vi "DAQmx(AI).TestLauncher.vi"() -> ()   [LabVIEW 2019, in "DAQmx(AI).lvclass"]
doc: "JKI State Machine Objects (SMO) 1.0.0.5\nJKI - JKI\nCopyright (c) 2016, JKI"
uses:
  DAQmx(AI).lvclass
  Typedefs/Scaling(MapRange)--Cluster.ctl
  Typedefs/InputConfiguration--Cluster.ctl
  Typedefs/Units -- Enum.ctl
  vi.lib/JKI/JKI SMO/SMO/Typedefs/SMOState --Enum.ctl
  C:/Users/Patrick/Documents/GitHub/Test (LV2019)/lv-venv/lv.lib/vi.lib/JKI/JKI SMO/SMO/SMO.lvclass
  Set Scaling (MapRange).vi
  vi.lib/JKI/JKI SMO/SMO/SMO.lvclass
panel:
  in  "TDMS File Path":path
  out "Waveform Chart":dbl(graph) caption="Waveform Graph"
  in  "Physical Channel":tag="SMO-Sim/ai0"
  out "Device Name":tag="SMO-Sim"
  out "Simulated":bool
  out "Device found":bool
  out "error out":errorcluster
  in  "Stop":bool
  # "Analog Input DAQmx Test Launcher"
  # "For instructions on how to use the JKI State Machine Objects, examples and video tutorials, visit:\nhttp://jki.net/state-machine-objects/\n\nJKI State Machine Objects™\nhttp://jki.net/state-machine-objects/\nCopyright (C) 2005-2016, JKI <info@jki.net>\nALL RIGHTS RESERVED"
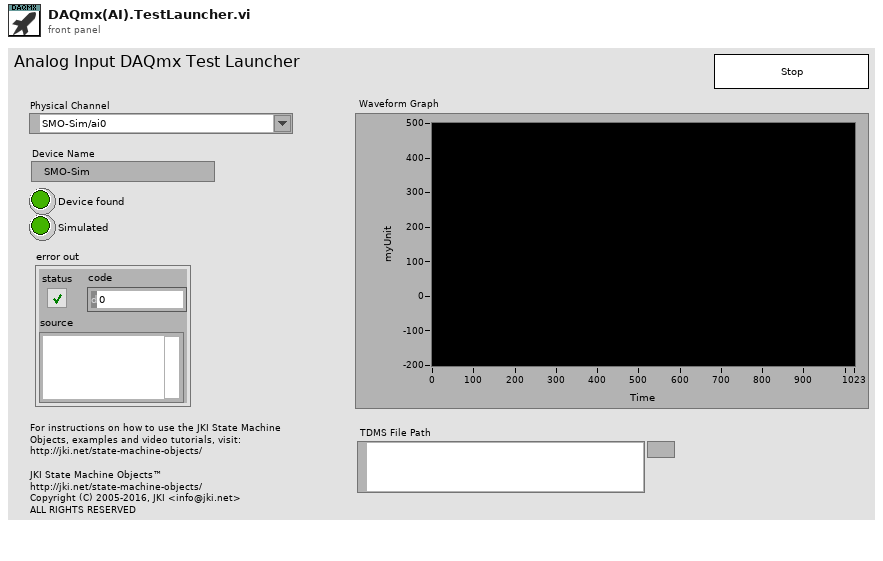
[diagram p1: front panel]
types:
  T1 = typedef "DAQmx(AI).lvclass/InputConfiguration--Cluster.ctl" = cluster{"input terminal":i32, "minimum value":dbl, "maximum value":dbl, "units":T2}
  T2 = typedef "DAQmx(AI).lvclass/Units -- Enum.ctl" = enum16{"Volts", "Amps", "Deg F", "Deg C", "Deg R", "Kelvins", "Strain", "Ohms", "Hz", "Seconds", "Meters", "Inches", "Degrees", "Radians", "Ticks", "g", "m/s^2", "m/s", "in/s", "Pascals", "Newtons", "Pounds", "kgf", "psi", "bar", "Nm", "oz-in", "lb-in", "lb-ft", "Volts/Volt", "mVolts/Volt", "From TEDS"}
  T3 = typedef "DAQmx(AI).lvclass/Scaling(MapRange)--Cluster.ctl" = cluster{"Minimum":dbl, "Maximum":dbl}
  T4 = typedef "DAQmx(AI).lvclass/PublicEvents--Cluster.ctl" = cluster{"Value Changed":refnum<user-event>, "Task Configuration":refnum<user-event>, "Scaling":refnum<user-event>}
  T5 = typedef "SMO.lvclass/Public Events.ctl" = cluster{"Error":refnum<user-event>, "State":refnum<user-event>, "Reserve State":refnum<user-event>}
  T6 = typedef "SMO.lvclass/SMOState --Enum.ctl" = enum16{"unknown", "Created", "Started", "Stopped"}
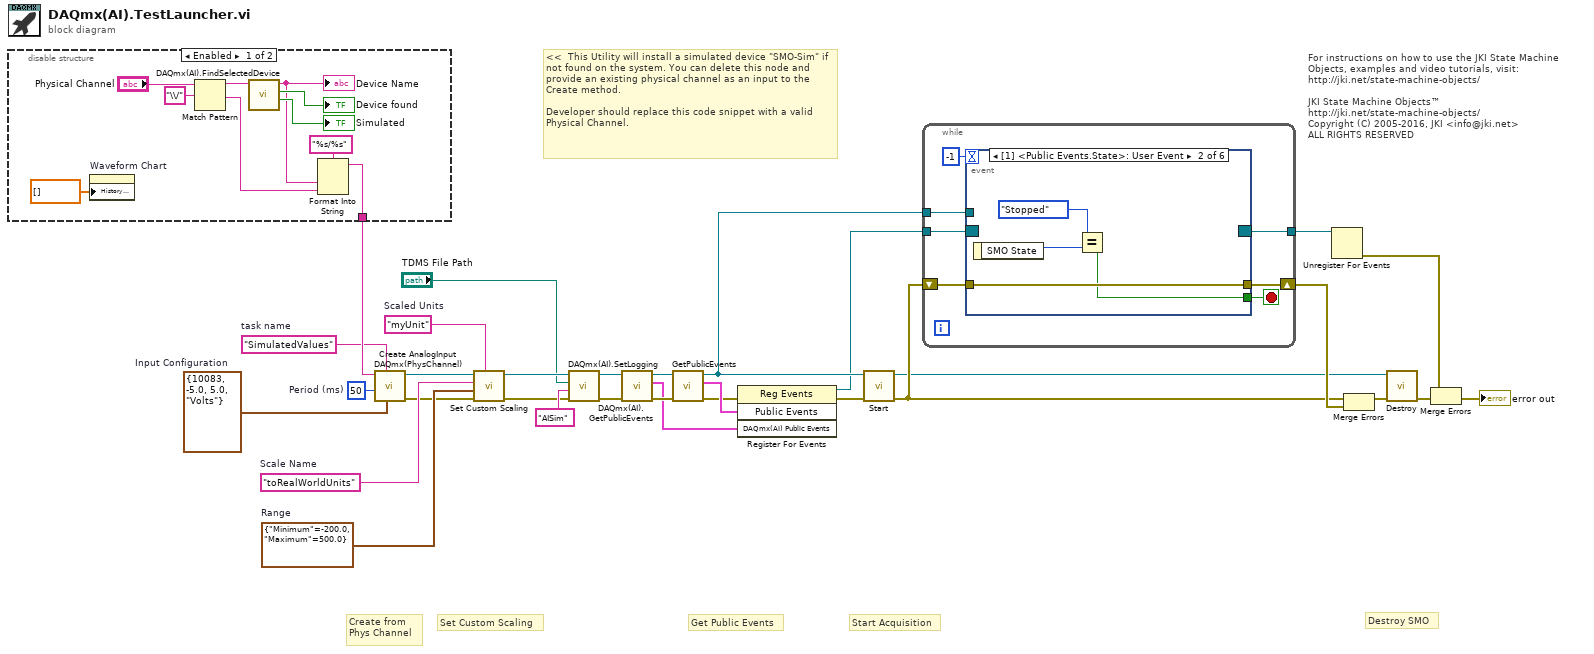
[diagram p0: block diagram]
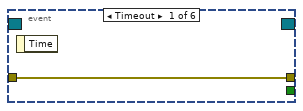
[diagram p3: hidden frame]
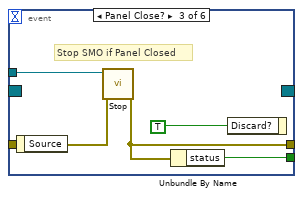
[diagram p4: hidden frame]
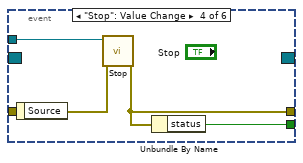
[diagram p5: hidden frame]
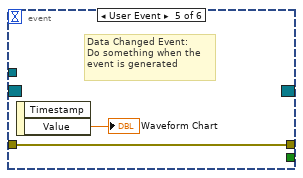
[diagram p6: hidden frame]
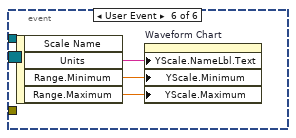
[diagram p7: hidden frame]
diagram:
  w1 = "SimulatedValues"  # task name
  w8 = T1 {"input terminal"=10083, "minimum value"=-5.0, "maximum value"=5.0, "units"=enum."Volts"}  # Input Configuration
  w9 = "myUnit"  # Scaled Units
  w11 = T3 {"Minimum"=-200.0, "Maximum"=500.0}  # Range
  w12 = "toRealWorldUnits"  # Scale Name
  w15 = i64 50  # Period (ms)
  # "Create from\nPhys Channel"
  # "Set Custom Scaling"
  # "<<  This Utility will install a simulated device \"SMO-Sim\" if not found on the system. You can delete this node and provide an existing physical channel as an input to the Create method.\n\nDeveloper should replace this code snippet with a valid Physical Channel."
  # "For instructions on how to use the JKI State Machine Objects, examples and video tutorials, visit:\nhttp://jki.net/state-machine-objects/\n\nJKI State Machine Objects™\nhttp://jki.net/state-machine-objects/\nCopyright (C) 2005-2016, JKI <info@jki.net>\nALL RIGHTS RESERVED"
  # "Get Public Events"
  # "Start Acquisition"
  # "Destroy SMO"
  n1 = disable-structure shown="Enabled" {
    disable-tunnel: [w33 _] -> w14
    frame Enabled {
      n2 = property on="Waveform Chart" class="WFChart (strict)"("History Data"=dbl[] []) -> ()  [unwired: 2 in, 2 out]
      n3 = Match Pattern(string="Physical Channel", regular expression="\\/") -> (before substring=w37:string, after substring=w35:string)  [unwired: 1 in, 2 out]
      n4 = call "DAQmx(AI).FindSelectedDevice.vi"("Device Name"=w37) -> ("Simulated"=→"Simulated":bool, "Device found"=→"Device found":bool, "ActiveDev"=w36:tag)  [unwired: 7 in, 1 out]
      "Device Name" <- w36
      n5 = Format Into String(format string="%s/%s", w36, w35) -> (resulting string=w33:string)  [unwired: 2 in, 1 out]
    }
    frame Disabled {
    }
  }
  n6 = call "Create AnalogInput DAQmx(PhysChannel).vi"("Input Configuration"=w8, "task name"=w1, "Period (ms)"=w15, "DAQmx Physical Channel"=w14) -> ("error out"=w10:errorcluster, "Subsystem out"=w13:refnum<class "DAQmx(AI).lvclass">)  [unwired: 5 in, 1 out]
  n7 = call-poly "Set Custom Scaling.vi"("Scaled Units"=w9, "error in (no error)"=w10, "Map Range"=w11, "Scale Name"=w12, "DAQmx(AI) in"=w13) -> ("error out"=w4:errorcluster, "DAQmx(AI) out"=w6:refnum<class "DAQmx(AI).lvclass">)  [unwired: 5 in]
  n8 = call "DAQmx(AI).SetLogging.vi"("error in (no error)"=w4, "Group Name"="AISim", "TDMS File Path"="TDMS File Path", "DAQmx(AI) in"=w6) -> ("error out"=w3:errorcluster, "DAQmx(AI) out"=w5:refnum<class "DAQmx(AI).lvclass">)  [unwired: 6 in]
  n9 = call "DAQmx(AI).GetPublicEvents.vi"("error in (no error)"=w3, "Subsystem"=w5) -> ("error out"=w18:errorcluster, "DAQmx(AI) Public Events"=w16:T4, "Subsystem out"=w17:refnum<class "DAQmx(AI).lvclass">)  [unwired: 7 in]
  n10 = call "GetPublicEvents.vi"("error in (no error)"=w18, "SMO"=w17) -> ("error out"=w20:errorcluster, "Public Events"=w21:T5, "SMO out"=w23:refnum<class "DAQmx(AI).lvclass">)  [unwired: 7 in]
  n11 = register-events(error in=w20, w21, w16) -> (reference out=w19:refnum<event-registration>, error out=w22:errorcluster)  [unwired: 1 in]
  n12 = call "Start.vi"("error in (no error)"=w22, "SMO"=w23) -> ("error out"=w26:errorcluster, "SMO out"=w24:refnum<class "DAQmx(AI).lvclass">)  [unwired: 8 in]
  n13 = while {
    shift-right: [w47] -> w30
    shift-left: w26 -> [w46]
    tunnel: w19 -> [w45]
    tunnel: [w44] -> w31
    tunnel: w23 -> [w43]
    stop <- w48 stop-if-true
    n14 = event shown="[1] <Public Events.State>: User Event" {
      selector: w45 -> [_ _ _ _ _ _]
      dyn-events: [_ _ _ _ _ _] -> w44
      timeout: -1 -> [_ _ _ _ _ _]
      tunnel: [_ w50 w54 w59 _ _] -> w48
      tunnel: w43 -> [_ _ w58 w62 _ _]
      tunnel: [w49 w53 w55 w60 w64 _] -> w47
      tunnel: w46 -> [w49 w53 w57 w61 w64 _]
      event Timeout {
        n15 = event-data() -> ()  [unwired: 1 in, 1 out]
      }
      event User Event {
        n16 = event-data() -> ("SMO State"=w52:T6)  [unwired: 1 in]
        n17 = Equal?(x=SMOState_--Enum."Stopped", y=w52) -> (x = y?=w50:bool)
      }
      event Panel Close? {
        # "Stop SMO if Panel Closed"
        n18 = event-data() -> ()  [unwired: 1 in, 1 out]
        n19 = call "Stop.vi"("error in (no error)"=w57, "SMO"=w58) -> ("error out"=w55:errorcluster)  [unwired: 8 in, 1 out]
        n20 = Unbundle By Name(w55) -> ("status"=w54:bool)
        n21 = event-data("Discard?"=TRUE ("OK")) -> ()  [unwired: 1 in, 1 out]
      }
      event "Stop": Value Change {
        n22 = event-data() -> ()  [unwired: 1 in, 1 out]
        n23 = call "Stop.vi"("error in (no error)"=w61, "SMO"=w62) -> ("error out"=w60:errorcluster)  [unwired: 8 in, 1 out]
        n24 = Unbundle By Name(w60) -> ("status"=w59:bool)
      }
      event User Event {
        # "Data Changed Event:\nDo something when the\nevent is generated"
        n25 = event-data() -> ("Value"=→"Waveform Chart":dbl)  [unwired: 1 in, 1 out]
      }
      event User Event {
        n26 = event-data() -> ("Units"=w67:string, "Range.Minimum"=w66:dbl, "Range.Maximum"=w65:dbl)  [unwired: 1 in, 1 out]
        n27 = property on="Waveform Chart" class="WFChart (strict)"("YScale.NameLbl.Text"=w67, "YScale.Minimum"=w66, "YScale.Maximum"=w65) -> ()  [unwired: 2 in, 2 out]
      }
    }
  }
  n28 = Unregister For Events(event registration refnum=w31) -> (error out=w29:errorcluster)  [unwired: 1 in]
  n29 = Merge Errors(w26, w30) -> (w25:errorcluster)
  n30 = call "Destroy.vi"("error in (no error)"=w25, "SMO"=w24) -> ("error out"=w27:errorcluster)  [unwired: 9 in]
  n31 = Merge Errors(w29, w27) -> (→"error out":errorcluster)
